vi "jMsg_TCPClient_Message_Send (create JSON).vi"(8 "error in (no error)":errorcluster, 10 "JSONPayload":refnum<class "JSONPayload.lvclass">, 11 "jMsg_TCPClient_Message_Send in":refnum<class "jMsg_TCPClient_Message_Send.lvclass">) -> (0 "error out":errorcluster, 3 "jMsg_TCPClient_Message_Send out":refnum<class "jMsg_TCPClient_Message_Send.lvclass">)   [LabVIEW 2019, in "jMsg_TCPClient_Message_Send.lvclass"]
uses:
  jMsg_TCPClient_Message_Send.lvclass
  JSONPacket/JSONPacket.lvclass
  <userlib>/Jet Engineering/JSMA/Libraries/jMsg Class/jMsg.lvclass
  C:/Program Files/National Instruments/LabVIEW 2019/user.lib/Jet Engineering/JSMA/Libraries/jMsg Class/jMsg.lvclass
  C:/projects/labview_multiplayer_snake/Main Codeline/Software/Code/Shared/TCP/TCPPacket/TCPPacket.lvclass
  JSONPayload/JSONPayload.lvclass
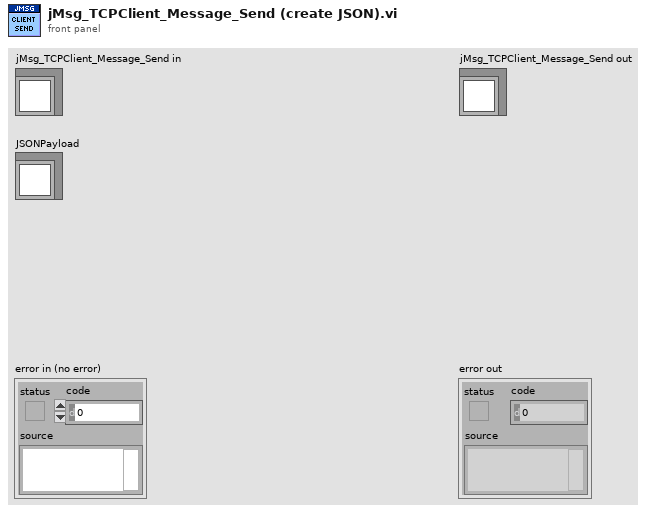
[diagram p1: front panel]
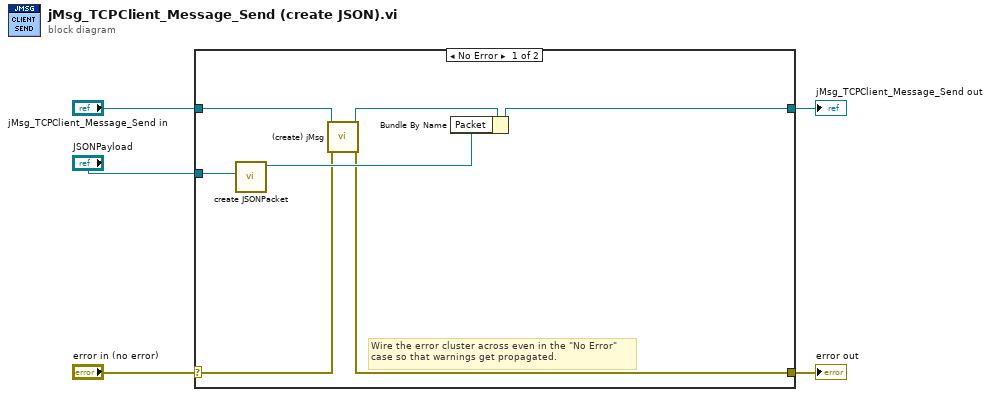
[diagram p0: block diagram]
diagram:
  n1 = case shown="No Error" "error in (no error)" {
    selector: "error in (no error)" -> [w7 w14]
    tunnel: [w6 w14] -> w4
    tunnel: [w11 w13] -> w2
    tunnel: "jMsg_TCPClient_Message_Send in" -> [w8 w13]
    tunnel: "JSONPayload" -> [w12 _]
    frame No Error {
      # "Wire the error cluster across even in the \"No Error\"\ncase so that warnings get propagated."
      n2 = call "create JSONPacket.vi"("JSONPayload"=w12) -> ("JSONPacket out"=w10:refnum<class "JSONPacket.lvclass">)  [unwired: 9 in, 1 out]
      n3 = call <userlib>:"(create) jMsg.vi"("error in (no error)"=w7, "jMsg in"=w8) -> ("error out"=w6:errorcluster, "jMsg out"=w9:refnum<class "jMsg_TCPClient_Message_Send.lvclass">)  [unwired: 8 in]
      n4 = Bundle By Name(cluster=w9, "Packet"=w10) -> (w11:refnum<class "jMsg_TCPClient_Message_Send.lvclass">)
    }
    frame Error {
    }
  }
  "error out" <- w4
  "jMsg_TCPClient_Message_Send out" <- w2
